vi "Pat Match Full with Move.vi"(0 "Minimum Match Score":sgl=500.0, 1 "Template File Path":path=path "C:/Users/Admin/Desktop/Main_Module_Assembly/Pattern recognition/templates/color.png", 5 "controller in":refnum<k24>, 11 "error in":errorcluster) -> (4 "Matched?":bool, 6 "Score":dbl, 8 "x rel move":dbl, 10 "y rel move":dbl, 15 "error out":errorcluster)   [LabVIEW 2011]
uses:
  C:/Users/Admin/Desktop/Gantry Code Transfer/source/Code Transfer/Aerotech.A3200.dll
  Aerotech.A3200.dll
  <vilib>/vision/driver/NI_Vision_Acquisition_Software.lvlib
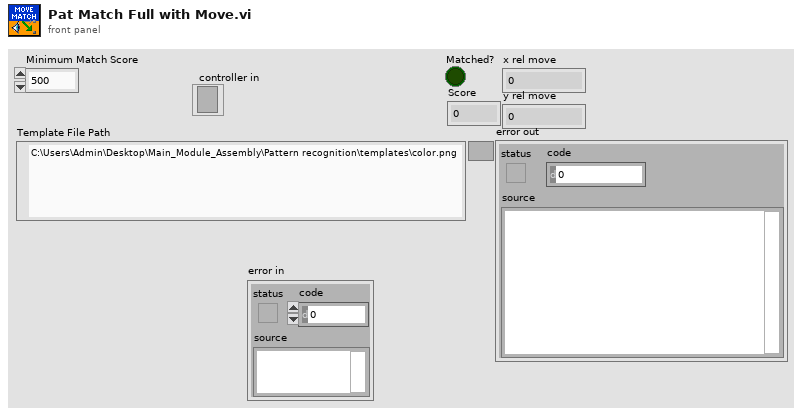
[diagram p1: front panel]
types:
  T1 = typedef "IMAQdx.ctl" = refnum<k21>
  T2 = typedef "IMAQ Image.ctl" = refnum<image>
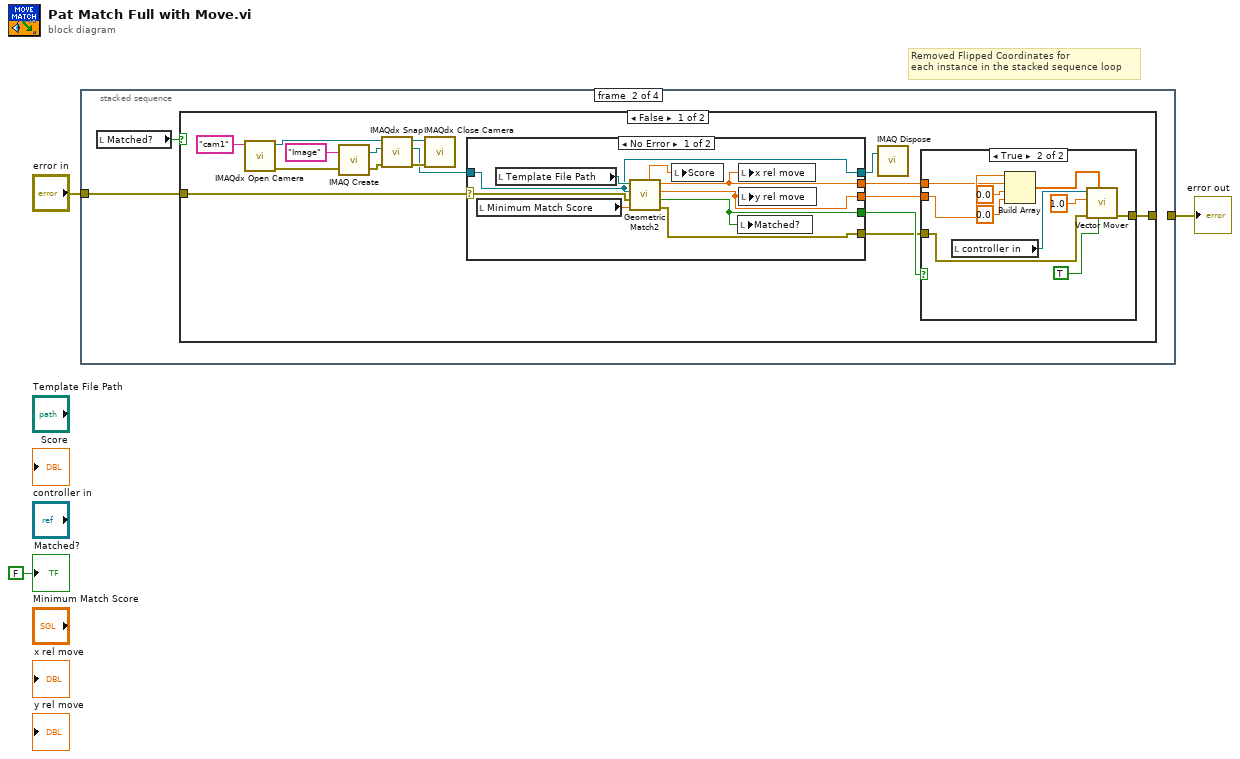
[diagram p0: block diagram]
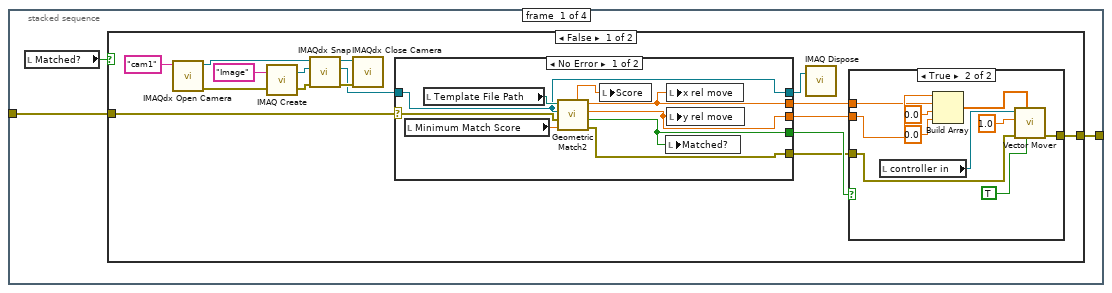
[diagram p2: hidden frame]
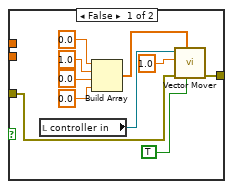
[diagram p3: hidden frame]
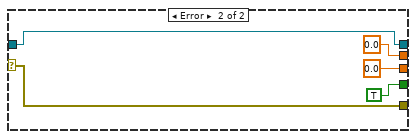
[diagram p4: hidden frame]
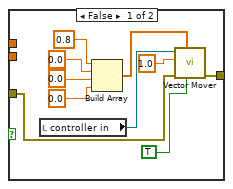
[diagram p6: hidden frame]
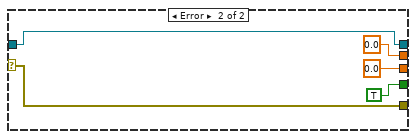
[diagram p7: hidden frame]
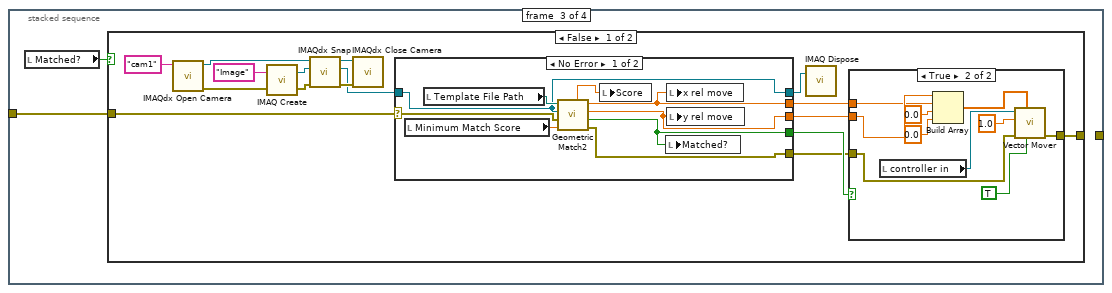
[diagram p9: hidden frame]
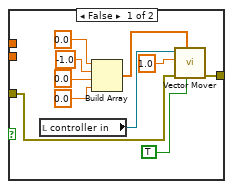
[diagram p10: hidden frame]
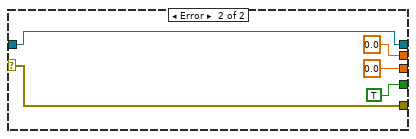
[diagram p11: hidden frame]
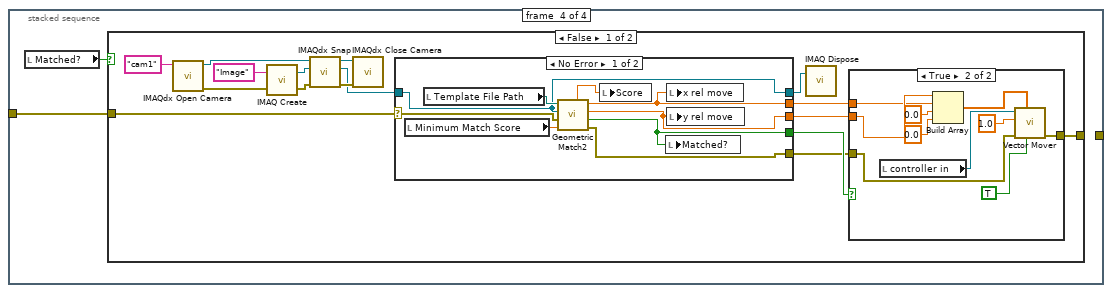
[diagram p13: hidden frame]
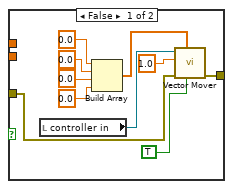
[diagram p14: hidden frame]
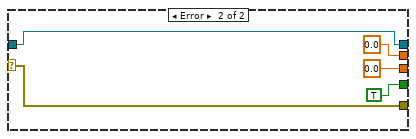
[diagram p15: hidden frame]
diagram:
  # "Removed Flipped Coordinates for \neach instance in the stacked sequence loop"
  n1 = stacked-sequence {
    tunnel: "error in" -> [w6 w59 w112 w165]
    tunnel: [w5 _ _ _] -> w3
    frame #0 {
      n2 = local read "Matched?"() -> (w4:bool)
      n3 = case shown="False" w4 {
        tunnel: w6 -> [w22 w57]
        tunnel: [w19 w57] -> w5
        frame False {
          n4 = call <vilib>:"IMAQdx Open Camera.vi"("Session In"="cam1" ("Interface Name")) -> ("error out"=w13:errorcluster, "Session Out"=w8:T1)  [unwired: 9 in]
          n5 = call "IMAQ Create"("Image Name"="Image", "error in (no error)"=w13) -> ("New Image"=w10:T2, "error out"=w9:errorcluster)  [unwired: 3 in]
          n6 = call <vilib>:"IMAQdx Snap.vi"("error in"=w9, "Image In"=w10, "Session In"=w8) -> ("error out"=w11:errorcluster, "Image Out"=w7:T2, "Session Out"=w12:T1)  [unwired: 6 in]
          n7 = call <vilib>:"IMAQdx Close Camera.vi"("error in"=w11, "Session In"=w12) -> ()  [unwired: 9 in, 1 out]
          n8 = case shown="No Error" w22 {
            selector: w22 -> [w50 w56]
            tunnel: [w51 w56] -> w20
            tunnel: [w44 TRUE ("Matched?")] -> w21
            tunnel: [w48 0.0 ("x rel move")] -> w18
            tunnel: [w47 0.0 ("y rel move")] -> w17
            tunnel: w7 -> [w43 w52]
            tunnel: [w43 w52] -> w16
            frame No Error {
              n9 = local read "Minimum Match Score"() -> (w45:sgl)
              n10 = local read "Template File Path"() -> (w46:path)
              n11 = call "Geometric Match2.vi"("Template File Path"=w46, "Image Src"=w43, "error in (no error)"=w50, "Minimum Match Score"=w45) -> ("Score"=w49:dbl, "x rel move"=w48:dbl, "y rel move"=w47:dbl, "Matched?"=w44:bool, "error out"=w51:errorcluster)
              n12 = local write "Score"(w49) -> ()
              n13 = local write "Matched?"(w44) -> ()
              n14 = local write "x rel move"(w48) -> ()
              n15 = local write "y rel move"(w47) -> ()
            }
            frame Error {
            }
          }
          n16 = call "IMAQ Dispose"("Image"=w16) -> ()  [unwired: 5 in, 1 out]
          n17 = case shown="True" w21 {
            tunnel: w20 -> [w30 w42]
            tunnel: [w25 w41] -> w19
            tunnel: w18 -> [_ w33]
            tunnel: w17 -> [_ w34]
            frame False {
              n18 = local read "controller in"() -> (w24:refnum<k24>)
              n19 = Build Array(0.0 ("element"), 1.0 ("element"), 0.0 ("element"), 0.0 ("element")) -> (w27:dbl[])
              n20 = call "Vector Mover.vi"("Absolute/Relative (F/T)"=TRUE, "Movement Vector"=w27, "error in (no error)"=w30, "Vector Speed"=1.0, "controller in"=w24) -> ("error out"=w25:errorcluster)  [unwired: 1 in, 3 out]
            }
            frame True {
              n21 = local read "controller in"() -> (w35:refnum<k24>)
              n22 = Build Array(w34, w33, 0.0 ("element"), 0.0 ("element")) -> (w36:dbl[])
              n23 = call "Vector Mover.vi"("Absolute/Relative (F/T)"=TRUE, "Movement Vector"=w36, "error in (no error)"=w42, "Vector Speed"=1.0, "controller in"=w35) -> ("error out"=w41:errorcluster)  [unwired: 1 in, 3 out]
            }
          }
        }
        frame True {
        }
      }
    }
    frame #1 {
      n24 = local read "Matched?"() -> (w58:bool)
      n25 = case shown="False" w58 {
        tunnel: w59 -> [w75 w110]
        tunnel: [w72 w110] -> _
        frame False {
          n26 = call <vilib>:"IMAQdx Open Camera.vi"("Session In"="cam1" ("Interface Name")) -> ("error out"=w66:errorcluster, "Session Out"=w61:T1)  [unwired: 9 in]
          n27 = call "IMAQ Create"("Image Name"="Image", "error in (no error)"=w66) -> ("New Image"=w63:T2, "error out"=w62:errorcluster)  [unwired: 3 in]
          n28 = call <vilib>:"IMAQdx Snap.vi"("error in"=w62, "Image In"=w63, "Session In"=w61) -> ("error out"=w64:errorcluster, "Image Out"=w60:T2, "Session Out"=w65:T1)  [unwired: 6 in]
          n29 = call <vilib>:"IMAQdx Close Camera.vi"("error in"=w64, "Session In"=w65) -> ()  [unwired: 9 in, 1 out]
          n30 = case shown="No Error" w75 {
            selector: w75 -> [w103 w109]
            tunnel: [w104 w109] -> w73
            tunnel: [w97 TRUE ("Matched?")] -> w74
            tunnel: [w101 0.0 ("x rel move")] -> w71
            tunnel: [w100 0.0 ("y rel move")] -> w70
            tunnel: w60 -> [w96 w105]
            tunnel: [w96 w105] -> w69
            frame No Error {
              n31 = local read "Minimum Match Score"() -> (w98:sgl)
              n32 = local read "Template File Path"() -> (w99:path)
              n33 = call "Geometric Match2.vi"("Template File Path"=w99, "Image Src"=w96, "error in (no error)"=w103, "Minimum Match Score"=w98) -> ("Score"=w102:dbl, "x rel move"=w101:dbl, "y rel move"=w100:dbl, "Matched?"=w97:bool, "error out"=w104:errorcluster)
              n34 = local write "Score"(w102) -> ()
              n35 = local write "Matched?"(w97) -> ()
              n36 = local write "x rel move"(w101) -> ()
              n37 = local write "y rel move"(w100) -> ()
            }
            frame Error {
            }
          }
          n38 = call "IMAQ Dispose"("Image"=w69) -> ()  [unwired: 5 in, 1 out]
          n39 = case shown="True" w74 {
            tunnel: w73 -> [w83 w95]
            tunnel: [w77 w94] -> w72
            tunnel: w71 -> [_ w86]
            tunnel: w70 -> [_ w87]
            frame False {
              n40 = local read "controller in"() -> (w76:refnum<k24>)
              n41 = Build Array(0.8 ("element"), 0.0 ("element"), 0.0 ("element"), 0.0 ("element")) -> (w80:dbl[])
              n42 = call "Vector Mover.vi"("Absolute/Relative (F/T)"=TRUE, "Movement Vector"=w80, "error in (no error)"=w83, "Vector Speed"=1.0, "controller in"=w76) -> ("error out"=w77:errorcluster)  [unwired: 1 in, 3 out]
            }
            frame True {
              n43 = local read "controller in"() -> (w89:refnum<k24>)
              n44 = Build Array(w87, w86, 0.0 ("element"), 0.0 ("element")) -> (w88:dbl[])
              n45 = call "Vector Mover.vi"("Absolute/Relative (F/T)"=TRUE, "Movement Vector"=w88, "error in (no error)"=w95, "Vector Speed"=1.0, "controller in"=w89) -> ("error out"=w94:errorcluster)  [unwired: 1 in, 3 out]
            }
          }
        }
        frame True {
        }
      }
    }
    frame #2 {
      n46 = local read "Matched?"() -> (w111:bool)
      n47 = case shown="False" w111 {
        tunnel: w112 -> [w128 w163]
        tunnel: [w125 w163] -> _
        frame False {
          n48 = call <vilib>:"IMAQdx Open Camera.vi"("Session In"="cam1" ("Interface Name")) -> ("error out"=w119:errorcluster, "Session Out"=w114:T1)  [unwired: 9 in]
          n49 = call "IMAQ Create"("Image Name"="Image", "error in (no error)"=w119) -> ("New Image"=w116:T2, "error out"=w115:errorcluster)  [unwired: 3 in]
          n50 = call <vilib>:"IMAQdx Snap.vi"("error in"=w115, "Image In"=w116, "Session In"=w114) -> ("error out"=w117:errorcluster, "Image Out"=w113:T2, "Session Out"=w118:T1)  [unwired: 6 in]
          n51 = call <vilib>:"IMAQdx Close Camera.vi"("error in"=w117, "Session In"=w118) -> ()  [unwired: 9 in, 1 out]
          n52 = case shown="No Error" w128 {
            selector: w128 -> [w156 w162]
            tunnel: [w157 w162] -> w126
            tunnel: [w150 TRUE ("Matched?")] -> w127
            tunnel: [w154 0.0 ("x rel move")] -> w124
            tunnel: [w153 0.0 ("y rel move")] -> w123
            tunnel: w113 -> [w149 w158]
            tunnel: [w149 w158] -> w122
            frame No Error {
              n53 = local read "Minimum Match Score"() -> (w151:sgl)
              n54 = local read "Template File Path"() -> (w152:path)
              n55 = call "Geometric Match2.vi"("Template File Path"=w152, "Image Src"=w149, "error in (no error)"=w156, "Minimum Match Score"=w151) -> ("Score"=w155:dbl, "x rel move"=w154:dbl, "y rel move"=w153:dbl, "Matched?"=w150:bool, "error out"=w157:errorcluster)
              n56 = local write "Score"(w155) -> ()
              n57 = local write "Matched?"(w150) -> ()
              n58 = local write "x rel move"(w154) -> ()
              n59 = local write "y rel move"(w153) -> ()
            }
            frame Error {
            }
          }
          n60 = call "IMAQ Dispose"("Image"=w122) -> ()  [unwired: 5 in, 1 out]
          n61 = case shown="True" w127 {
            tunnel: w126 -> [w136 w148]
            tunnel: [w130 w147] -> w125
            tunnel: w124 -> [_ w139]
            tunnel: w123 -> [_ w140]
            frame False {
              n62 = local read "controller in"() -> (w129:refnum<k24>)
              n63 = Build Array(0.0 ("element"), -1.0 ("element"), 0.0 ("element"), 0.0 ("element")) -> (w133:dbl[])
              n64 = call "Vector Mover.vi"("Absolute/Relative (F/T)"=TRUE, "Movement Vector"=w133, "error in (no error)"=w136, "Vector Speed"=1.0, "controller in"=w129) -> ("error out"=w130:errorcluster)  [unwired: 1 in, 3 out]
            }
            frame True {
              n65 = local read "controller in"() -> (w141:refnum<k24>)
              n66 = Build Array(w140, w139, 0.0 ("element"), 0.0 ("element")) -> (w142:dbl[])
              n67 = call "Vector Mover.vi"("Absolute/Relative (F/T)"=TRUE, "Movement Vector"=w142, "error in (no error)"=w148, "Vector Speed"=1.0, "controller in"=w141) -> ("error out"=w147:errorcluster)  [unwired: 1 in, 3 out]
            }
          }
        }
        frame True {
        }
      }
    }
    frame #3 {
      n68 = local read "Matched?"() -> (w164:bool)
      n69 = case shown="False" w164 {
        tunnel: w165 -> [w181 w216]
        tunnel: [w178 w216] -> _
        frame False {
          n70 = call <vilib>:"IMAQdx Open Camera.vi"("Session In"="cam1" ("Interface Name")) -> ("error out"=w172:errorcluster, "Session Out"=w167:T1)  [unwired: 9 in]
          n71 = call "IMAQ Create"("Image Name"="Image", "error in (no error)"=w172) -> ("New Image"=w169:T2, "error out"=w168:errorcluster)  [unwired: 3 in]
          n72 = call <vilib>:"IMAQdx Snap.vi"("error in"=w168, "Image In"=w169, "Session In"=w167) -> ("error out"=w170:errorcluster, "Image Out"=w166:T2, "Session Out"=w171:T1)  [unwired: 6 in]
          n73 = call <vilib>:"IMAQdx Close Camera.vi"("error in"=w170, "Session In"=w171) -> ()  [unwired: 9 in, 1 out]
          n74 = case shown="No Error" w181 {
            selector: w181 -> [w209 w215]
            tunnel: [w210 w215] -> w179
            tunnel: [w203 TRUE ("Matched?")] -> w180
            tunnel: [w207 0.0 ("x rel move")] -> w177
            tunnel: [w206 0.0 ("y rel move")] -> w176
            tunnel: w166 -> [w202 w211]
            tunnel: [w202 w211] -> w175
            frame No Error {
              n75 = local read "Minimum Match Score"() -> (w204:sgl)
              n76 = local read "Template File Path"() -> (w205:path)
              n77 = call "Geometric Match2.vi"("Template File Path"=w205, "Image Src"=w202, "error in (no error)"=w209, "Minimum Match Score"=w204) -> ("Score"=w208:dbl, "x rel move"=w207:dbl, "y rel move"=w206:dbl, "Matched?"=w203:bool, "error out"=w210:errorcluster)
              n78 = local write "Score"(w208) -> ()
              n79 = local write "Matched?"(w203) -> ()
              n80 = local write "x rel move"(w207) -> ()
              n81 = local write "y rel move"(w206) -> ()
            }
            frame Error {
            }
          }
          n82 = call "IMAQ Dispose"("Image"=w175) -> ()  [unwired: 5 in, 1 out]
          n83 = case shown="True" w180 {
            tunnel: w179 -> [w189 w201]
            tunnel: [w183 w200] -> w178
            tunnel: w177 -> [_ w192]
            tunnel: w176 -> [_ w193]
            frame False {
              n84 = local read "controller in"() -> (w182:refnum<k24>)
              n85 = Build Array(0.0 ("element"), 0.0 ("element"), 0.0 ("element"), 0.0 ("element")) -> (w186:dbl[])
              n86 = call "Vector Mover.vi"("Absolute/Relative (F/T)"=TRUE, "Movement Vector"=w186, "error in (no error)"=w189, "Vector Speed"=1.0, "controller in"=w182) -> ("error out"=w183:errorcluster)  [unwired: 1 in, 3 out]
            }
            frame True {
              n87 = local read "controller in"() -> (w194:refnum<k24>)
              n88 = Build Array(w193, w192, 0.0 ("element"), 0.0 ("element")) -> (w195:dbl[])
              n89 = call "Vector Mover.vi"("Absolute/Relative (F/T)"=TRUE, "Movement Vector"=w195, "error in (no error)"=w201, "Vector Speed"=1.0, "controller in"=w194) -> ("error out"=w200:errorcluster)  [unwired: 1 in, 3 out]
            }
          }
        }
        frame True {
        }
      }
    }
  }
  "error out" <- w3
  "Matched?" <- FALSE ("Matched?")
